vi "mini auto 1.vi"   [LabVIEW 2014]
uses:
  Support Files/Global Data!!!.vi
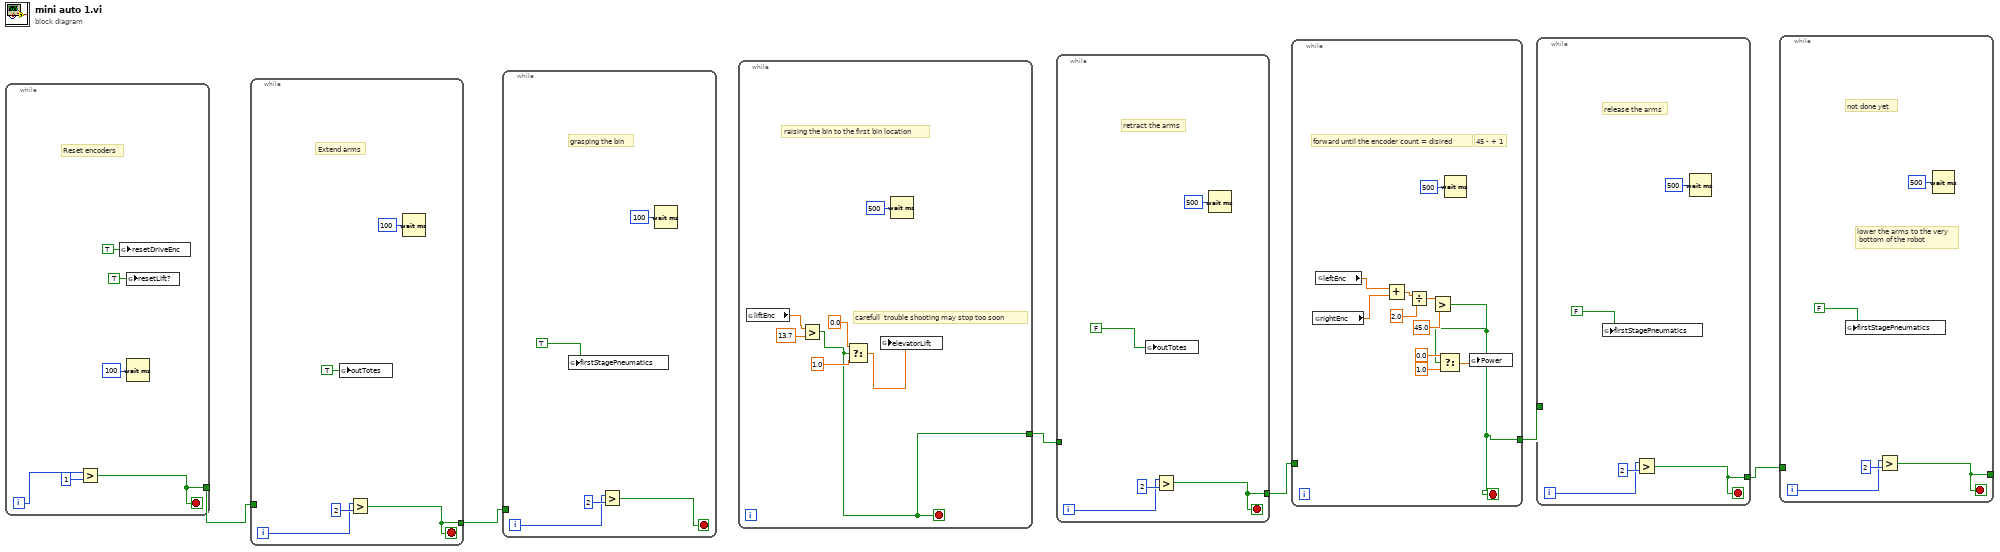
[diagram p0: block diagram]
diagram:
  n1 = while {
    tunnel: [w9] -> w6
    i -> [w11]
    stop <- w9 stop-if-true
    # "Reset encoders"
    n2 = Greater?(x=w11, y=1) -> (0:w9:bool)
    n3 = global write "Global Data!!!.vi" "resetDriveEnc"(TRUE ("resetDriveEnc")) -> ()
    n4 = global write "Global Data!!!.vi" "resetLift?"(TRUE ("resetLift?")) -> ()
    n5 = Wait (ms)(milliseconds to wait=u32 100) -> ()  [unwired: 1 out]
  }
  n6 = while {
    tunnel: w6 -> [_]
    tunnel: [w13] -> w5
    i -> [w14]
    stop <- w13 stop-if-true
    # "Extend arms"
    n7 = global write "Global Data!!!.vi" "outTotes"(TRUE ("outTotes")) -> ()
    n8 = Greater?(x=w14, y=2) -> (0:w13:bool)
    n9 = Wait (ms)(milliseconds to wait=u32 100) -> ()  [unwired: 1 out]
  }
  n10 = while {
    tunnel: w5 -> [_]
    i -> [w19]
    stop <- w18 stop-if-true
    # "grasping the bin"
    n11 = global write "Global Data!!!.vi" "firstStagePneumatics"(TRUE ("outTotes")) -> ()
    n12 = Greater?(x=w19, y=2) -> (0:w18:bool)
    n13 = Wait (ms)(milliseconds to wait=u32 100) -> ()  [unwired: 1 out]
  }
  n14 = while {
    tunnel: [w23] -> w4
    stop <- w23 stop-if-true
    # "carefull  trouble shooting may stop too soon"
    # "raising the bin to the first bin location"
    n15 = global read "Global Data!!!.vi" "liftEnc"() -> (w25:dbl)
    n16 = Greater?(x=w25, y=13.7) -> (0:w23:bool)
    n17 = Select(t=0.0, s=w23, f=1.0) -> (s? t:f=w24:dbl)
    n18 = global write "Global Data!!!.vi" "elevatorLift"(w24) -> ()
    n19 = Wait (ms)(milliseconds to wait=u32 500) -> ()  [unwired: 1 out]
  }
  n20 = while {
    tunnel: w4 -> [_]
    tunnel: [w30] -> w3
    i -> [w31]
    stop <- w30 stop-if-true
    # "retract the arms"
    n21 = global write "Global Data!!!.vi" "outTotes"(FALSE ("outTotes")) -> ()
    n22 = Greater?(x=w31, y=2) -> (0:w30:bool)
    n23 = Wait (ms)(milliseconds to wait=u32 500) -> ()  [unwired: 1 out]
  }
  n24 = while {
    tunnel: w3 -> [_]
    tunnel: [w35] -> w2
    stop <- w35 stop-if-true
    # "45 - + 1"
    # "forward until the encoder count = disired"
    n25 = global read "Global Data!!!.vi" "rightEnc"() -> (w44:dbl)
    n26 = global read "Global Data!!!.vi" "leftEnc"() -> (w43:dbl)
    n27 = Add(x=w43, y=w44) -> (x+y=w42:dbl)
    n28 = Divide(x=w42, y=2.0) -> (x/y=w40:dbl)
    n29 = Greater?(x=w40, y=45.0) -> (0:w35:bool)
    n30 = Select(t=0.0, s=w35, f=1.0) -> (s? t:f=w36:dbl)
    n31 = Wait (ms)(milliseconds to wait=u32 500) -> ()  [unwired: 1 out]
    n32 = global write "Global Data!!!.vi" "Power"(w36) -> ()
  }
  n33 = while {
    tunnel: [w46] -> w1
    tunnel: w2 -> [_]
    i -> [w47]
    stop <- w46 stop-if-true
    # "release the arms"
    n34 = global write "Global Data!!!.vi" "firstStagePneumatics"(FALSE ("outTotes")) -> ()
    n35 = Greater?(x=w47, y=2) -> (0:w46:bool)
    n36 = Wait (ms)(milliseconds to wait=u32 500) -> ()  [unwired: 1 out]
  }
  n37 = while {
    tunnel: [w51] -> _
    tunnel: w1 -> [_]
    i -> [w52]
    stop <- w51 stop-if-true
    # "lower the arms to the very\n bottom of the robot"
    # "not done yet"
    n38 = global write "Global Data!!!.vi" "firstStagePneumatics"(FALSE ("outTotes")) -> ()
    n39 = Greater?(x=w52, y=2) -> (0:w51:bool)
    n40 = Wait (ms)(milliseconds to wait=u32 500) -> ()  [unwired: 1 out]
  }
